vi "If Position Available.vi"(4 "column":i32, 6 "row":i32, 9 "available white position":i32[][](array[numeric]), 10 "available black position":i32[][](array[numeric]), 11 "current color":T1) -> (1 "found?":bool)   [LabVIEW 2011, in "Othello.xctl"]
uses:
  Othello.xctl
  Control/Pict Ring Chess.ctl
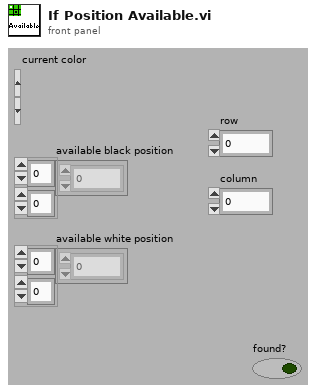
[diagram p1: front panel]
types:
  T1 = typedef "Othello.xctl/Pict Ring Chess.ctl" = u16
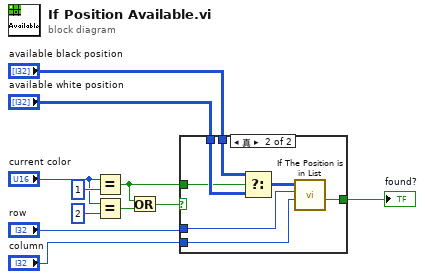
[diagram p0: block diagram]
diagram:
  n1 = Equal?(x="current color", y=T1 1) -> (x = y?=w3:bool)
  n2 = Equal?(x="current color", y=T1 2) -> (x = y?=w2:bool)
  n3 = Or(x=w3, y=w2) -> (x .or. y?=w1:bool)
  n4 = case shown="真" w1 {
    tunnel: "available white position" -> [_ w18]
    tunnel: "available black position" -> [_ w17]
    tunnel: "column" -> [_ w16]
    tunnel: "row" -> [_ w15]
    tunnel: [_ w14] -> w7
    tunnel: w3 -> [_ w12]
    frame False {
    }
    frame True {
      n5 = Select(t=w17, s=w12, f=w18) -> (s? t:f=w13:i32[][])
      n6 = call "If The Position is in List.vi"("column"=w16, "row"=w15, "available position"=w13) -> ("found?"=w14:bool)  [unwired: 8 out]
    }
  }
  "found?" <- w7
